vi "Queue Nested Status.vi"(11 "jettl Event Actor in":refnum<class "jettl Event Actor.lvclass">) -> (0 "Queue Nested Count":i32, 1 "Queue Nested Aliases":string[](array[string]), 2 "Any Exist?":bool)   [LabVIEW 2021, in "jettl.lvlib" / "jettl Event Actor.lvlib" / "jettl Event Actor.lvclass"]
uses:
  jettl Event Actor.lvclass
  jettl Event Actor.lvclass/jettl Event Actor.ctl
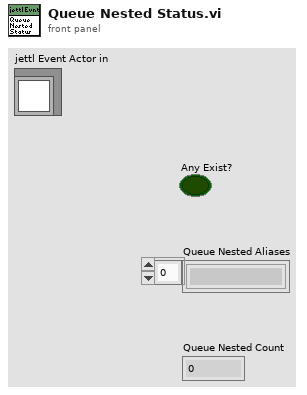
[diagram p1: front panel]
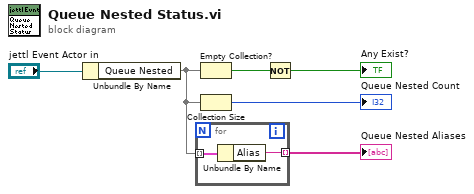
[diagram p0: block diagram]
diagram:
  n1 = Unbundle By Name("jettl Event Actor in") -> ("Queue Nested"=w6:map{string, refnum<data-value>})
  n2 = for {
    tunnel: [w7] -> w1 mode=indexing
    tunnel: w6 -> [w8] mode=indexing
    n3 = Unbundle By Name(w8) -> ("Alias"=w7:string)
  }
  "Queue Nested Aliases" <- w1
  n4 = Empty Collection?(1:w6) -> (0:w5:bool)
  n5 = Collection Size(1:w6) -> (0:→"Queue Nested Count":i32)
  n6 = Not(x=w5) -> (.not. x?=→"Any Exist?":bool)
